vi "Root path.vi"(8 "error in":errorcluster) -> (0 "Error Out":errorcluster, 3 "Root Path's":cluster{"Sub vi's":path, "Authentication":path})   [LabVIEW 2022 SP3]
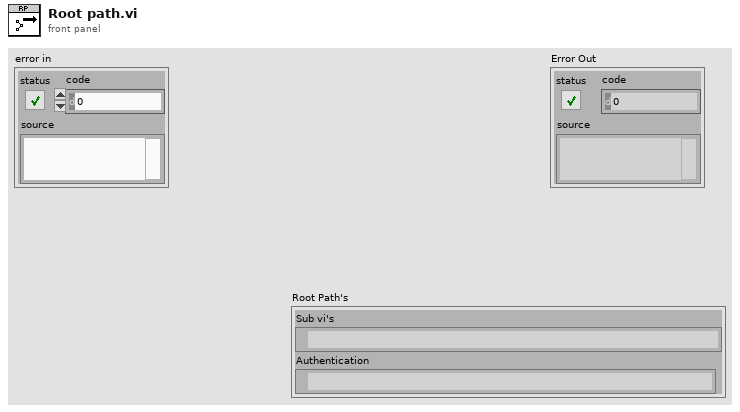
[diagram p1: front panel]
types:
  T1 = enum32{"invalid app kind", "Development System", "Run Time System", "Student Edition", "Embedded LabVIEW", "Evaluation", "Custom"}
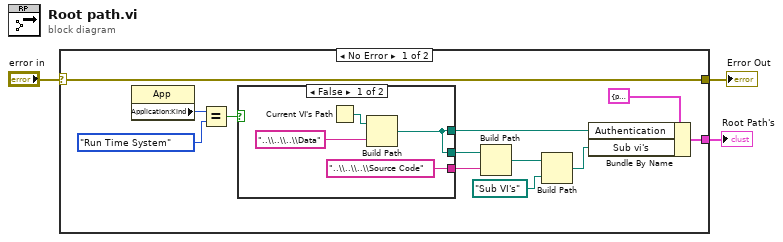
[diagram p0: block diagram]
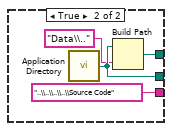
[diagram p2: hidden frame]
diagram:
  n1 = case shown="No Error" "error in" {
    selector: "error in" -> [w12 w24]
    tunnel: [w12 w24] -> w2
    tunnel: [w11 _] -> w1
    frame No Error {
      n2 = property class="App"() -> ("Application:Kind"=w15:T1)  [unwired: 2 in, 2 out]
      n3 = Equal?(x=w15, y=T1."Run Time System") -> (x = y?=w13:bool)
      n4 = case shown="False" w13 {
        tunnel: ["..\\..\\..\\Source Code" ("name or relative path") "..\\..\\..\\..\\Source Code" ("name or relative path")] -> w10
        tunnel: [w16 w22] -> w7
        tunnel: [w16 w21] -> w6
        frame False {
          n5 = Current VI's Path() -> (path=w17:path)
          n6 = Build Path(base path=w17, name or relative path="..\\..\\..\\Data") -> (appended path=w16:path)
        }
        frame True {
          n7 = call <vilib>:"Application Directory.vi"() -> ("Application Directory"=w21:path)
          n8 = Build Path(base path=w21, name or relative path="Data\\..") -> (appended path=w22:path)
        }
      }
      n9 = Build Path(base path=w6, name or relative path=w10) -> (appended path=w9:path)
      n10 = Build Path(base path=w9, name or relative path=path "Sub VI's") -> (appended path=w5:path)
      n11 = Bundle By Name(cluster=cluster{"Sub vi's":path, "Authentication":path} {"Sub vi's"=path "", "Authentication"=path ""} ("Cluster"), "Authentication"=w7, "Sub vi's"=w5) -> (w11:cluster{"Sub vi's":path, "Authentication":path})
    }
    frame Error {
    }
  }
  "Error Out" <- w2
  "Root Path's" <- w1
